vi "m1m3_getSample_FPGAData.vi"(8 "error in (no error)":errorcluster, 11 "FPGAData_Ctl":T1={"Timestamp"=0.0, "ModbusTxInternalFIFOOverflow[5]"=[FALSE, FALSE, FALSE, FALSE, FALSE], "ModbusInvalidInstruction[5]"=[FALSE, FALSE, FALSE, FALSE, FALSE], "ModbusWaitForRxFrameTimeout[5]"=[FALSE, FALSE, FALSE, FALSE, FALSE], "ModbusStartBitError[5]"=[FALSE, FALSE, FALSE, FALSE, FALSE], "ModbusStopBitError[5]"=[FALSE, FALSE, FALSE, FALSE, FALSE], "ModbusRxDataFIFOOverflow[5]"=[FALSE, FALSE, FALSE, FALSE, FALSE], "ModbusTxByteCount[5]"=[0, 0, 0, 0, 0], "ModbusTxFrameCount[5]"=[0, 0, 0, 0, 0], "ModbusRxByteCount[5]"=[0, 0, 0, 0, 0], "ModbusRxFrameCount[5]"=[0, 0, 0, 0, 0], "FPGATime"=0.0}) -> (0 "error out":errorcluster, 2 "function return":i32, 3 "FPGAData_Ctl out":T1)   [LabVIEW 2016, in "SALLV_m1m3.lvlib"]
doc: "int m1m3_shm_getSample_FPGADataLV(m1m3_FPGADataLV *FPGAData_Ctl );"
uses:
  SALLV_m1m3.lvlib
  DataTypes/FPGAData.ctl
  SALLV_m1m3.so
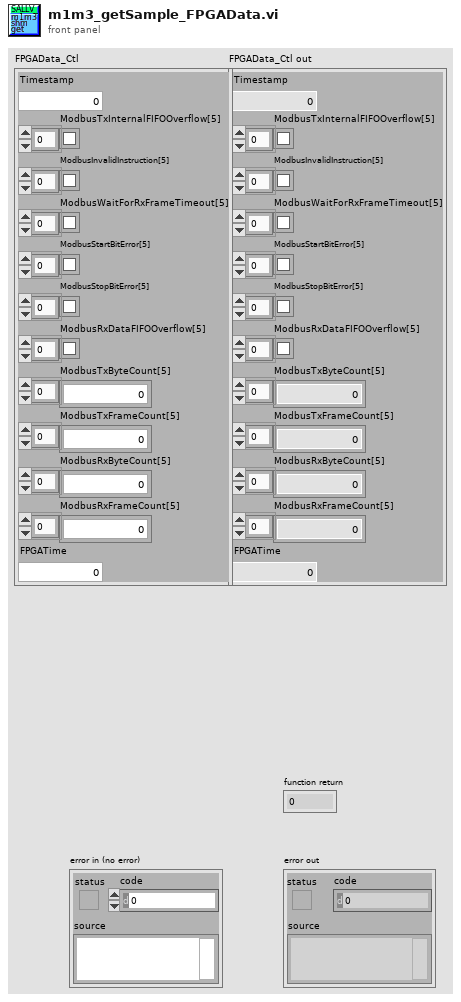
[diagram p1: front panel]
types:
  T1 = typedef "SALLV_m1m3.lvlib/FPGAData.ctl" = cluster{"Timestamp":dbl, "ModbusTxInternalFIFOOverflow[5]":bool[], "ModbusInvalidInstruction[5]":bool[], "ModbusWaitForRxFrameTimeout[5]":bool[], "ModbusStartBitError[5]":bool[], "ModbusStopBitError[5]":bool[], "ModbusRxDataFIFOOverflow[5]":bool[], "ModbusTxByteCount[5]":u32[], "ModbusTxFrameCount[5]":u32[], "ModbusRxByteCount[5]":u32[], "ModbusRxFrameCount[5]":u32[], "FPGATime":dbl}
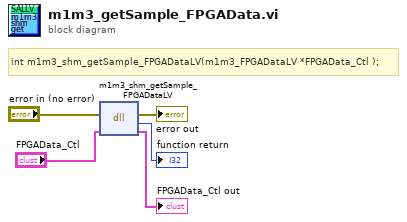
[diagram p0: block diagram]
diagram:
  # "int m1m3_shm_getSample_FPGADataLV(m1m3_FPGADataLV *FPGAData_Ctl );"
  n1 = dll-call lib="opt/CODE/ts_m1m3supporteui/SALLV_m1m3/SALLV_m1m3.*" fn="m1m3_shm_getSample_FPGADataLV"(error in="error in (no error)", "FPGAData_Ctl"="FPGAData_Ctl") -> (error out=→"error out":errorcluster, →"function return":i32, "FPGAData_Ctl"=→"FPGAData_Ctl out":T1)  [unwired: 2 in, 1 out]
